vi "Const frame c keyword.vi"() -> (3 "Const frame c keyword":string[](array[string]))   [LabVIEW 2018, in "Frame Analizer.lvclass"]
uses:
  Frame Analizer.lvclass
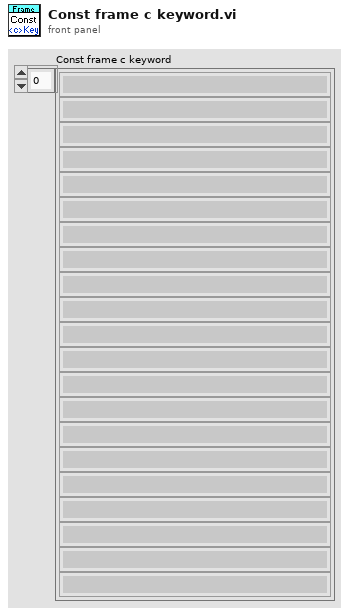
[diagram p1: front panel]
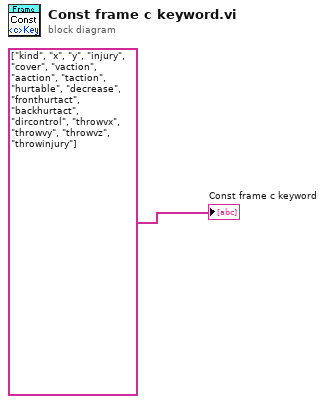
[diagram p0: block diagram]
diagram:
  "Const frame c keyword" <- string[] ["kind", "x", "y", "injury", "cover", "vaction", "aaction", "taction", "hurtable", "decrease", "fronthurtact", "backhurtact", "dircontrol", "throwvx", "throwvy", "throwvz", "throwinjury"]
